vi "host.vi"() -> ()   [LabVIEW 2015]
panel:
  in  "IC":enum16{"IS61WV5128", "IS61WV25616"}(ring)
  in  "State":enum16{"Reading data ", "Writing data"}(ring)
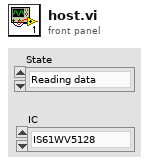
[diagram p1: front panel]
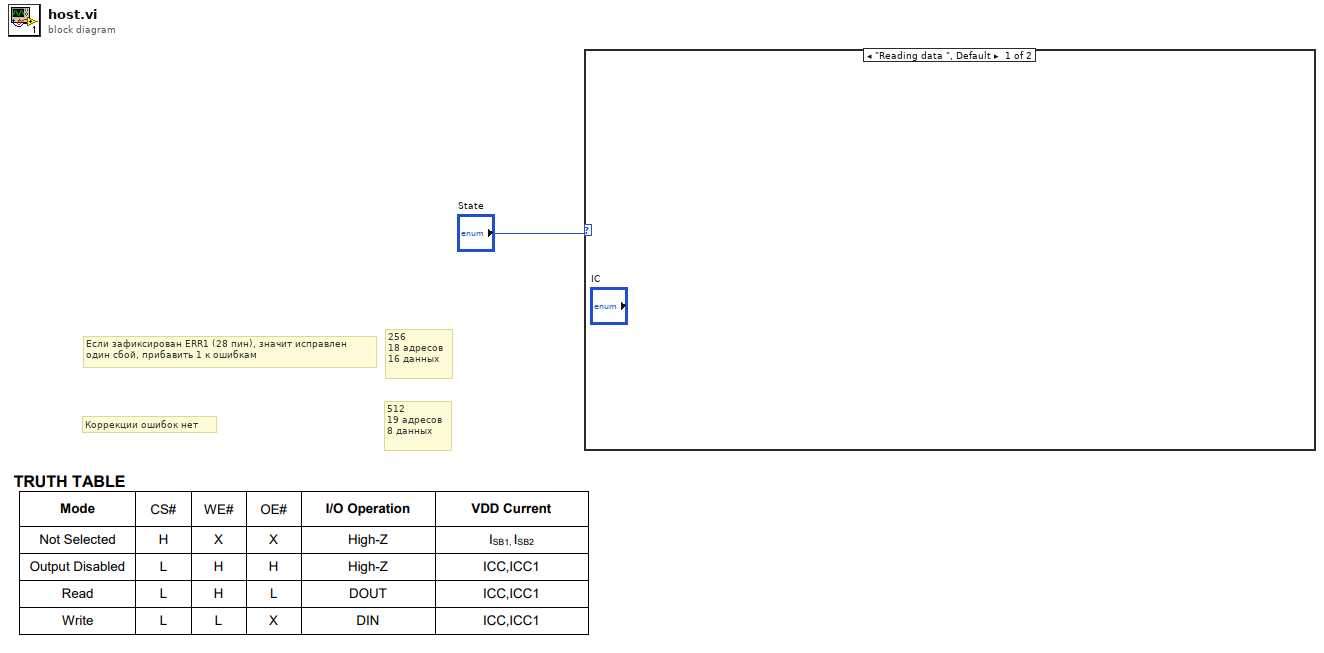
[diagram p0: block diagram]
diagram:
  # "Коррекции ошибок нет"
  # "Если зафиксирован ERR1 (28 пин), значит исправлен\nодин сбой, прибавить 1 к ошибкам"
  # "256\n18 адресов\n16 данных"
  # "512\n19 адресов\n8 данных"
  n1 = case shown="\"Reading data \", Default" "State" {
    frame "Reading data ", Default {
    }
    frame "Writing data" {
    }
  }
